vi "Get Calculated Cash Stats.vi"(11 "Cash Stats":T2) -> (3 "Calculated Cash Stats":T1)   [LabVIEW 2021]
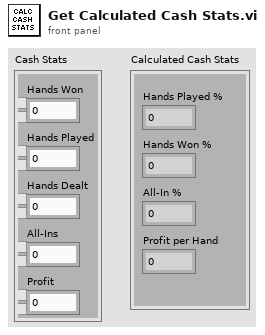
[diagram p1: front panel]
types:
  T1 = cluster{"Hands Played %":dbl, "Hands Won %":dbl, "All-In %":dbl, "Profit per Hand":dbl}
  T2 = cluster{"Hands Won":u32, "Hands Played":u32, "Hands Dealt":u32, "All-Ins":u32, "Profit":dbl}
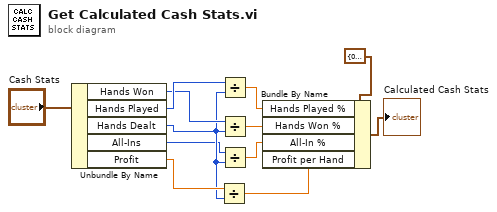
[diagram p0: block diagram]
diagram:
  n1 = Unbundle By Name("Cash Stats") -> ("Hands Won"=w8:u32, "Hands Played"=w9:u32, "Hands Dealt"=w3:u32, "All-Ins"=w2:u32, "Profit"=w5:dbl)
  n2 = Divide(x=w5, y=w3) -> (x/y=w6:dbl)
  n3 = Divide(x=w9, y=w3) -> (x/y=w10:dbl)
  n4 = Divide(x=w8, y=w3) -> (x/y=w11:dbl)
  n5 = Divide(x=w2, y=w3) -> (x/y=w4:dbl)
  n6 = Bundle By Name(cluster=T1 {"Hands Played %"=0.0, "Hands Won %"=0.0, "All-In %"=0.0, "Profit per Hand"=0.0} ("Calculated Cash Stats"), "Hands Played %"=w10, "Hands Won %"=w11, "All-In %"=w4, "Profit per Hand"=w6) -> (→"Calculated Cash Stats":T1)
